vi "messageDefinitionParse.vi"(2 "New String":string, 3 "Body":string, 4 "Constants":string) -> (0 "Body Out":string, 1 "Constants Out":string)   [LabVIEW 2012]
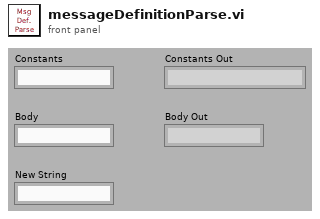
[diagram p1: front panel]
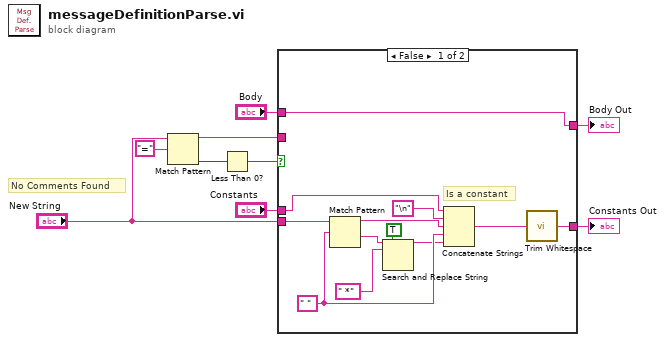
[diagram p0: block diagram]
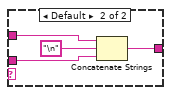
[diagram p3: hidden frame]
diagram:
  # "No Comments Found"
  n1 = Match Pattern(string="New String", regular expression="=") -> (before substring=w4:string, offset past match=w2:i32)  [unwired: 1 in, 2 out]
  n2 = Less Than 0?(x=w2) -> (x < 0?=w3:bool)
  n3 = case shown="False" w3 {
    tunnel: w4 -> [_ w22]
    tunnel: "New String" -> [w16 _]
    tunnel: "Constants" -> [w21 w23]
    tunnel: [w18 w23] -> w9
    tunnel: "Body" -> [w20 w25]
    tunnel: [w20 w24] -> w8
    frame False {
      w11 = " " ("regular expression")
      # "Is a constant"
      n4 = Match Pattern(string=w16, regular expression=w11) -> (before substring=w12:string, after substring=w15:string)  [unwired: 1 in, 2 out]
      n5 = Search and Replace String(replace all?=TRUE ("replace all? (F)"), input string=w15, search string=" *") -> (result string=w10:string)  [unwired: 5 in, 3 out]
      n6 = Concatenate Strings(w21, "\n" ("string"), w12, w11, w10) -> (w17:string)
      n7 = call <vilib>:"Trim Whitespace.vi"("string"=w17) -> ("trimmed string"=w18:string)  [unwired: 1 in]
    }
    frame True {
      # "Not a Constant"
      n8 = case shown="\"\", \" \"" w22 {
        tunnel: w25 -> [w26 w30]
        tunnel: [w26 w29] -> w24
        tunnel: w22 -> [_ w28]
        frame "", " " {
        }
        frame Default {
          n9 = Concatenate Strings(w30, "\n" ("string"), w28) -> (w29:string)
        }
      }
    }
  }
  "Constants Out" <- w9
  "Body Out" <- w8
